vi "Stop.vi"() -> ()   [LabVIEW 2014]
panel:
  out "Stop":bool
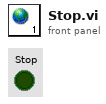
[diagram p1: front panel]
diagram:
